vi "Teardown Example.vi"(8 "error in (no error)":errorcluster, 11 "Module Was Already Running?":bool) -> (0 "error out":errorcluster)   [LabVIEW 2023]
uses:
  DeviceManager/DeviceManager.lvlib
panel:
  # "Connector Pane"
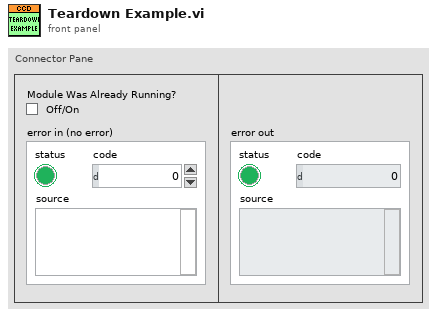
[diagram p1: front panel]
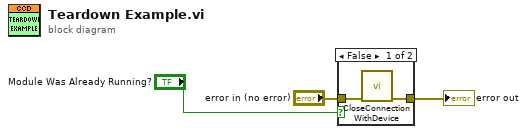
[diagram p0: block diagram]
diagram:
  n1 = case shown="False" "Module Was Already Running?" {
    tunnel: [w5 w6] -> w1
    tunnel: "error in (no error)" -> [w4 w6]
    frame False {
      n2 = call "CloseConnectionWithDevice.vi"("error in (no error)"=w4) -> ("error out"=w5:errorcluster)  [unwired: 10 in]
    }
    frame True {
    }
  }
  "error out" <- w1
